vi "Newport ITX-D3N Extract Data.vi"(8 "Error In":errorcluster, 11 "TCP String Data":string) -> (0 "Error Out":errorcluster, 1 "Add to Array":bool, 2 "Relative Humidity":dbl, 3 "Temperature":dbl)   [LabVIEW 2016]
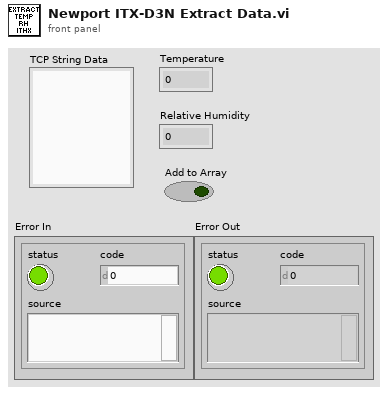
[diagram p1: front panel]
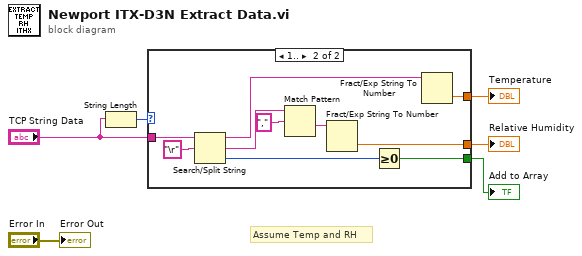
[diagram p0: block diagram]
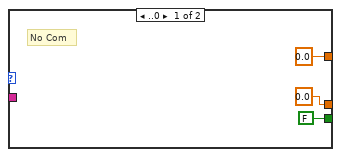
[diagram p2: hidden frame]
diagram:
  # "Assume Temp and RH"
  n1 = String Length(string="TCP String Data") -> (length=w2:i32)
  n2 = case shown="1.." w2 {
    tunnel: "TCP String Data" -> [_ w18]
    tunnel: [FALSE w17] -> w5
    tunnel: [0.0 w14] -> w3
    tunnel: [0.0 w13] -> w4
    frame ..0 {
      # "No Com"
    }
    frame 1.. {
      n3 = Search/Split String(string=w18, search string/char (-)="\r") -> (substring before match=w15:string, match + rest of string=w11:string, offset of match=w16:i32)  [unwired: 1 in]
      n4 = Match Pattern(string=w11, regular expression="," ("search string/char (-)")) -> (after substring=w12:string)  [unwired: 1 in, 3 out]
      n5 = Fract/Exp String To Number(string=w12) -> (number=w13:dbl)  [unwired: 3 in, 1 out]
      n6 = Greater Or Equal To 0?(x=w16) -> (x >= 0?=w17:bool)
      n7 = Fract/Exp String To Number(string=w15) -> (number=w14:dbl)  [unwired: 3 in, 1 out]
    }
  }
  "Add to Array" <- w5
  "Relative Humidity" <- w4
  "Temperature" <- w3
  "Error Out" <- "Error In"
